vi "PressureSensorTest.vi"() -> ()   [LabVIEW 2013]
uses:
  PressureSensorAction.ctl
  <vilib>/Rock Robotics/SystemInterfaces/Typedef/FPGA_TypedefAnalogModule.ctl
  <vilib>/Rock Robotics/SystemInterfaces/AI/FPGA_AIChannel.ctl
panel:
  out "Pressure":dbl
  in  "PressureScaler":dbl=1.0
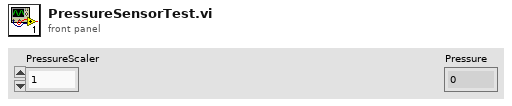
[diagram p1: front panel]
types:
  T1 = typedef "FPGA_AIChannel.ctl" = enum8{"AI 1", "AI 2", "AI 3", "AI 4", "AI 5", "AI 6", "AI 7", "AI 8", "Invalid"}
  T2 = typedef "FPGA_TypedefAnalogModule.ctl" = enum16{"Analog Module 1", "Analog Module 2"}
  T3 = typedef "PressureSensorAction.ctl" = enum16{"Init", "ReadValue", "Disable"}
  T4 = typedef "WPI_AnalogChannelDevRef.ctl" = cluster{"DevStatus":errorcluster, "Analog Module":T2, "Analog Channel":T1}
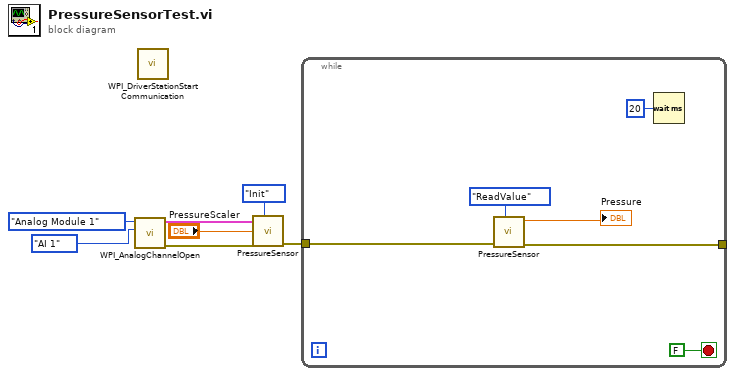
[diagram p0: block diagram]
diagram:
  n1 = call <vilib>:"WPI_AnalogChannelOpen.vi"("Analog Channel"=FPGA_AIChannel."AI 1", "Analog Module (Module 1)"=FPGA_TypedefAnalogModule."Analog Module 1") -> ("error out"=w3:errorcluster, "AIDeviceRef"=w6:T4)  [unwired: 8 in]
  n2 = call <vilib>:"WPI_DriverStationStart Communication.vi"() -> ()  [unwired: 12 in]
  n3 = call "PressureSensor.vi"("Action"=PressureSensorAction."Init", "error in (no error)"=w3, "PressureScaler"="PressureScaler", "AIDeviceRef"=w6) -> ("error out"=w1:errorcluster)  [unwired: 6 in, 1 out]
  n4 = while {
    tunnel: w1 -> [w11]
    tunnel: [w10] -> _
    stop <- FALSE stop-if-true
    n5 = call "PressureSensor.vi"("Action"=PressureSensorAction."ReadValue", "error in (no error)"=w11) -> ("error out"=w10:errorcluster, "Pressure"=→"Pressure":dbl)  [unwired: 8 in]
    n6 = Wait (ms)(milliseconds to wait=u32 20) -> ()  [unwired: 1 out]
  }
